vi "resampling.vi"() -> ()   [LabVIEW 2020]
uses:
  <vilib>/Analysis/3filter.llb/Filter Passband Type.ctl
  <vilib>/Analysis/2dsp.llb/Real FFT.vi
  <vilib>/Analysis/2dsp.llb/Decimate (single shot, DBL).vi
  <vilib>/Analysis/2dsp.llb/Upsample (DBL).vi
  <vilib>/Analysis/3filter.llb/Butterworth Filter (DBL).vi
  <vilib>/Analysis/NI_AALBase.lvlib
  <vilib>/Analysis/NI_AALPro.lvlib
panel:
  in  "STOP":bool
  out "Frequency content of the input and the output":waveform(dbl)[](graph)
  out "Time content of the input and the output":waveform(dbl)[](graph)
  in  "FFT size":i32=-1
  in  "Sampling frequency":dbl=1.0
  in  "Frequency":dbl=0.0078125 format="%0.4e"
  in  "Samples":i32=128
  in  "Decimating factor":dbl
  in  "Upsampling factor":dbl
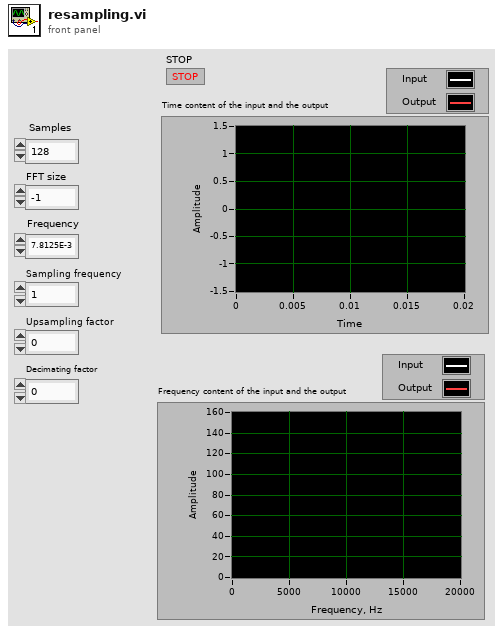
[diagram p1: front panel]
types:
  T1 = typedef "NI_AALBase.lvlib/Filter Passband Type.ctl" = enum32{"Lowpass", "Highpass", "Bandpass", "Bandstop"}
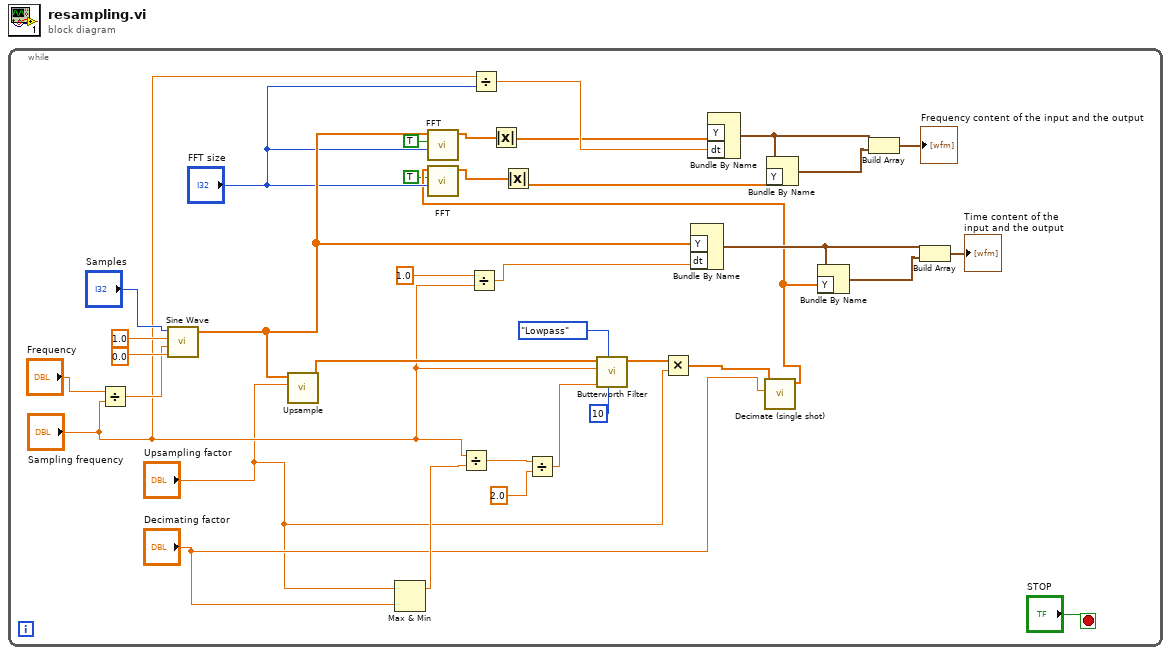
[diagram p0: block diagram]
diagram:
  n1 = while {
    stop <- "STOP" stop-if-true
    n2 = Divide(x="Frequency", y="Sampling frequency") -> (x/y=w25:dbl)
    n3 = call <vilib>:"Sine Wave.vi"("samples"="Samples", "amplitude"=1.0, "frequency"=w25, "phase in"=0.0) -> ("sine wave"=w23:dbl[])  [unwired: 1 in, 2 out]
    n4 = call-poly <vilib>:"Upsample.vi"("upsampling factor"="Upsampling factor", "X"=w23) -> ("Upsampled Array"=w30:dbl[])  [unwired: 8 in, 1 out]
    n5 = Max & Min(x="Upsampling factor", y="Decimating factor") -> (max(x,y)=w24:dbl)  [unwired: 1 out]
    n6 = call-poly <vilib>:"FFT.vi"("FFT size"="FFT size", "shift?"=TRUE, "X"=w23) -> ("FFT {X}"=w16:cdb[])  [unwired: 7 in, 1 out]
    n7 = Divide(x="Sampling frequency", y=w24) -> (x/y=w34:dbl)
    n8 = Divide(x=1.0, y="Sampling frequency") -> (x/y=w21:dbl)
    n9 = Divide(x="Sampling frequency", y="FFT size") -> (x/y=w18:dbl)
    n10 = Absolute Value(x=w16) -> (abs(x)=w15:dbl[])
    n11 = Divide(x=w34, y=2.0) -> (x/y=w31:dbl)
    n12 = call-poly <vilib>:"Butterworth Filter.vi"("order"=10, "filter type"=Filter_Passband_Type."Lowpass", "low cutoff freq: fl"=w31, "sampling freq: fs"="Sampling frequency", "X"=w30) -> ("Filtered X"=w33:dbl[])  [unwired: 3 in, 1 out]
    n13 = Multiply(x=w33, y="Upsampling factor") -> (x*y=w6:dbl[])
    n14 = Bundle By Name("Y"=w23, "dt"=w21) -> (w8:waveform(dbl))  [unwired: 1 in]
    n15 = Bundle By Name("Y"=w15, "dt"=w18) -> (w11:waveform(dbl))  [unwired: 1 in]
    n16 = call-poly <vilib>:"Decimate (single shot).vi"("decimating factor"="Decimating factor", "X"=w6) -> ("Decimated Array"=w4:dbl[])  [unwired: 8 in, 1 out]
    n17 = call-poly <vilib>:"FFT.vi"("FFT size"="FFT size", "shift?"=TRUE, "X"=w4) -> ("FFT {X}"=w14:cdb[])  [unwired: 7 in, 1 out]
    n18 = Absolute Value(x=w14) -> (abs(x)=w13:dbl[])
    n19 = Bundle By Name(cluster=w11, "Y"=w13) -> (w12:waveform(dbl))
    n20 = Bundle By Name(cluster=w8, "Y"=w4) -> (w9:waveform(dbl))
    n21 = Build Array(w11, w12) -> (→"Frequency content of the input and the output":waveform(dbl)[])
    n22 = Build Array(w8, w9) -> (→"Time content of the input and the output":waveform(dbl)[])
  }
